vi "Set Parameter.vi"(8 "error in (no error)":errorcluster, 10 "Analyze Parameter":refnum<class "Analyze Parameter Base.lvclass">, 11 "Analyze Compound Analysis Base in":refnum<class "Analyze Compound Analysis Base.lvclass">) -> (0 "error out":errorcluster, 3 "Analyze Compound Analysis Base out":refnum<class "Analyze Compound Analysis Base.lvclass">)   [LabVIEW 2020, in "Analyze.lvlib" / "Analyze Compound Analysis Base.lvclass"]
uses:
  Analyze Compound Analysis Base.lvclass
  Analyze Parameter/Analyze Parameter Base/Analyze Parameter Base.lvclass
  Analyze Compound Analysis Base.lvclass/Analyze Compound Analysis Base.ctl
  Analyze BaseClass/Analyze BaseClass/Analyze BaseClass.lvclass
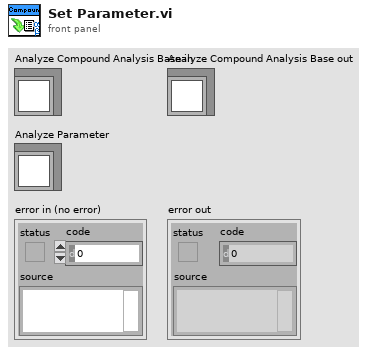
[diagram p1: front panel]
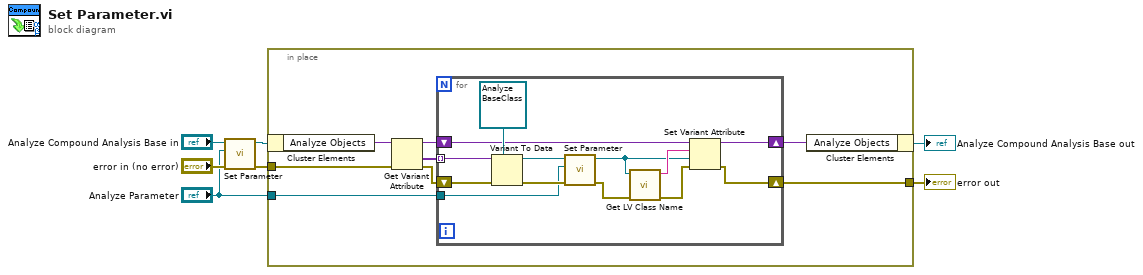
[diagram p0: block diagram]
diagram:
  n1 = call-parent "Set Parameter.vi"("error in (no error)"="error in (no error)", "Analyze Parameter"="Analyze Parameter", "Analyze BaseClass in"="Analyze Compound Analysis Base in") -> ("error out"=w4:errorcluster, "Analyze BaseClass out"=w5:refnum<class "Analyze Compound Analysis Base.lvclass">)  [unwired: 7 in]
  n2 = in-place {
    in-place-border: w4 -> [w9]
    in-place-border: [w13] -> w1
    in-place-border: "Analyze Parameter" -> [w11]
    n3 = in-place-cluster #1(w5) -> ("Analyze Objects"=w15:variant)
    n4 = Get Variant Attribute(Variant=w15, error in=w9) -> (duplicate Variant=w12:variant, values=w14:variant[], error out=w8:errorcluster)  [unwired: 2 in, 1 out]
    n5 = for {
      tunnel: w14 -> [w27] mode=indexing
      shift-right: [w22] -> w13
      shift-left: w8 -> [w26]
      shift-right: [w24] -> w10
      shift-left: w12 -> [w25]
      tunnel: w11 -> [w18]
      n6 = Variant To Data(error in=w26, type=refnum<class "Analyze BaseClass.lvclass"> refnum ("Analyze.lvlib:Analyze BaseClass.lvlib:Analyze BaseClass.lvclass"), Variant=w27) -> (data=w20:refnum<class "Analyze BaseClass.lvclass">, error out=w19:errorcluster)
      n7 = call-dynamic "Set Parameter.vi"("error in (no error)"=w19, "Analyze Parameter"=w18, "Analyze BaseClass in"=w20) -> ("error out"=w16:errorcluster, "Analyze BaseClass out"=w17:refnum<class "Analyze BaseClass.lvclass">)  [unwired: 7 in]
      n8 = call <vilib>:"Get LV Class Name.vi"("error in (no error)"=w16, "object"=w17) -> ("error out"=w23:errorcluster, "class name"=w21:string)  [unwired: 8 in]
      n9 = Set Variant Attribute(Variant=w25, name=w21, value=w17, error in=w23) -> (Variant out=w24:variant, error out=w22:errorcluster)  [unwired: 1 out]
    }
    n10 = in-place-cluster #1("Analyze Objects"=w10) -> (→"Analyze Compound Analysis Base out":refnum<class "Analyze Compound Analysis Base.lvclass">)
  }
  "error out" <- w1
